vi "Main.vi"   [LabVIEW 2021]
uses:
  Dev Actor/Dev Actor/Dev Actor.lvclass
  C:/Program Files/National Instruments/LabVIEW 2021/vi.lib/jettl/jettl/Actor/Actor/Actor.lvclass
  <vilib>/jettl/jettl/jettl/jettl/jettl.lvclass
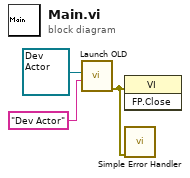
[diagram p0: block diagram]
diagram:
  n1 = call <vilib>:"Launch OLD.vi"("Alias"="Dev Actor", "Actor"=refnum<class "Dev Actor.lvclass"> refnum ("Process.lvlib:Process.lvclass")) -> ("error out"=w1:errorcluster)  [unwired: 9 in]
  n2 = invoke class="VI" method="FP.Close"(error in=w1) -> ()  [unwired: 2 in, 3 out]
  n3 = call <vilib>:"Simple Error Handler.vi"("error in (no error)"=w1) -> ()  [unwired: 4 in, 5 out]
